vi "Do.vi"(8 "error in (no error)":errorcluster, 10 "Actor in":refnum<class "Actor.lvclass">, 11 "Set Lengths Msg":refnum<class "Set Lengths Msg.lvclass">) -> (0 "error out":errorcluster, 2 "Actor out":refnum<class "Actor.lvclass">)   [LabVIEW 2020, in "BNT_DAQmx.lvlib" / "Set Lengths Msg.lvclass"]
doc: "This VI delivers the message to the actor by calling the appropriate method(s) on the actor."
uses:
  Set Lengths Msg.lvclass
  <vilib>/ActorFramework/Actor/Actor.lvclass
  C:/Users/holge/Documents/LVP/BNT/PGC/Packages/CSPP_Core/Messages/CSPP_PVUpdate Msg/CSPP_PVUpdate Msg.lvclass
  BNT_DAQmx-MCSV-DOPWM/BNT_DAQmx-MCSV-DOPWM.lvclass
  C:/Program Files (x86)/National Instruments/LabVIEW 2020/vi.lib/ActorFramework/Actor/Actor.lvclass
  CSPP_Core/Messages/CSPP_PVUpdate Msg/CSPP_PVUpdate Msg.lvclass/CSPP_PVUpdate Msg.ctl
  CSPP_Core/Classes/CSPP_ProcessVariables/ProcessVariable/PV.lvclass/PV.ctl
  Set Lengths Msg.lvclass/Set Lengths Msg.ctl
  CSPP_Core/Classes/CSPP_ProcessVariables/ProcessVariable/PV.lvclass
  CSPP_Core/Messages/CSPP_PVUpdate Msg/CSPP_PVUpdate Msg.lvclass
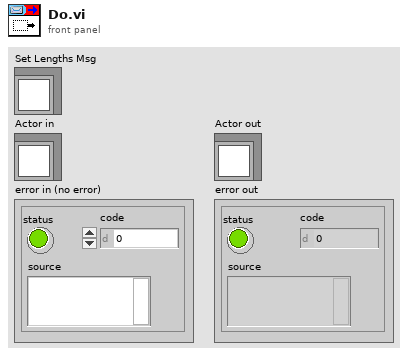
[diagram p1: front panel]
types:
  T1 = cluster{"PWM Lengths":dbl[unit][], "Start Index":i32}
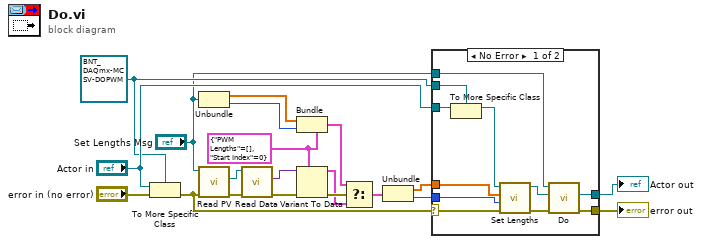
[diagram p0: block diagram]
diagram:
  w13 = T1 {"PWM Lengths"=[], "Start Index"=0} ("Type")
  w16 = refnum<class "BNT_DAQmx-MCSV-DOPWM.lvclass"> refnum ("Actor in")
  n1 = To More Specific Class(target class=w16, reference="Actor in", error in="error in (no error)") -> (error out=w10:errorcluster)  [unwired: 1 out]
  n2 = Unbundle ("Pre-Unbundler")("Set Lengths Msg") -> (w2:dbl[unit][], w1:i32)
  n3 = call "Read PV.vi"("error in (no error)"=w10, "CS++PVUpdate Msg in"="Set Lengths Msg") -> ("error out"=w15:errorcluster, "PV"=w12:refnum<class "PV.lvclass">)  [unwired: 7 in, 1 out]
  n4 = call "Read Data.vi"("error in (no error)"=w15, "PV in"=w12) -> ("error out"=w6:errorcluster, "Data"=w5:variant)  [unwired: 7 in, 1 out]
  n5 = Bundle ("Pre-Bundler")(cluster=w13, "PWM Lengths"=w2, "Start Index"=w1) -> (w7:T1)
  n6 = Variant To Data(error in=w6, type=w13, Variant=w5) -> (data=w8:T1, error out=w14:errorcluster)
  n7 = Select ("MainSelect")(t=w7, s=w14, f=w8) -> (s? t:f=w11:T1)
  n8 = Unbundle ("Main-Unbundler")(w11) -> ("PWM Lengths"=w4:dbl[unit][], "Start Index"=w3:i32)
  n9 = case shown="No Error" w10 {
    selector: w10 -> [w31 w33]
    tunnel: [w26 w33] -> w19
    tunnel: [w27 w32] -> w18
    tunnel: "Actor in" -> [w30 w32]
    tunnel: w16 -> [w29 _]
    tunnel: "Set Lengths Msg" -> [w23 _]
    tunnel: w4 -> [w22 _]
    tunnel: w3 -> [w21 _]
    frame No Error {
      n10 = To More Specific Class ("To More Specific Class (internal)")(target class=w29, reference=w30) -> (specific class reference=w28:refnum<class "BNT_DAQmx-MCSV-DOPWM.lvclass">)  [unwired: 1 in, 1 out]
      n11 = call "Set Lengths.vi"("error in"=w31, "Start Index"=w21, "PWM Lengths"=w22, "BNT_DAQmx-MCSV-DOPWM in"=w28) -> ("error out"=w25:errorcluster, "BNT_DAQmx-MCSV-DOPWM out"=w24:refnum<class "BNT_DAQmx-MCSV-DOPWM.lvclass">)  [unwired: 6 in]
      n12 = call-parent "Do.vi"("error in (no error)"=w25, "Actor in"=w24, "CS++PVUpdate Msg"=w23) -> ("error out"=w26:errorcluster, "Actor out"=w27:refnum<class "Actor.lvclass">)  [unwired: 7 in]
    }
    frame Error {
    }
  }
  "error out" <- w19
  "Actor out" <- w18
